vi "Read XML_Parse BC Acyclic Frames.vi"(8 "error in (no error)":errorcluster, 10 "channel in":T1, 11 ".NET Refnum in":refnum<k24>) -> (0 "error out":errorcluster, 2 "channel out":T1, 3 ".NET Refnum out":refnum<k24>)   [LabVIEW 2017, in "Ballard 1553 System Explorer.lvlib"]
uses:
  Ballard 1553 System Explorer.lvlib
  Ballard_Channel.ctl
  Ballard_BC.ctl
  Ballard_message.ctl
  Ballard_messageType.ctl
  Ballard_CWD1.ctl
  Ballard_CWD2.ctl
  Ballard_minorFrame.ctl
  Ballard_majorFrame.ctl
  Ballard_acyclicFrame.ctl
  Ballard_RT.ctl
  Ballard_RT subAddress.ctl
  Ballard_RT direction.ctl
  Ballard_RT rtMode.ctl
  Ballard_RT modeCode.ctl
  D:/Ballard-1553-Custom-Device Inline Async/Source/System Explorer/SubVIs/Parse XML Ballard/Ballard_BTI_XML_Deserializer.dll
  Ballard_BTI_XML_Deserializer.dll
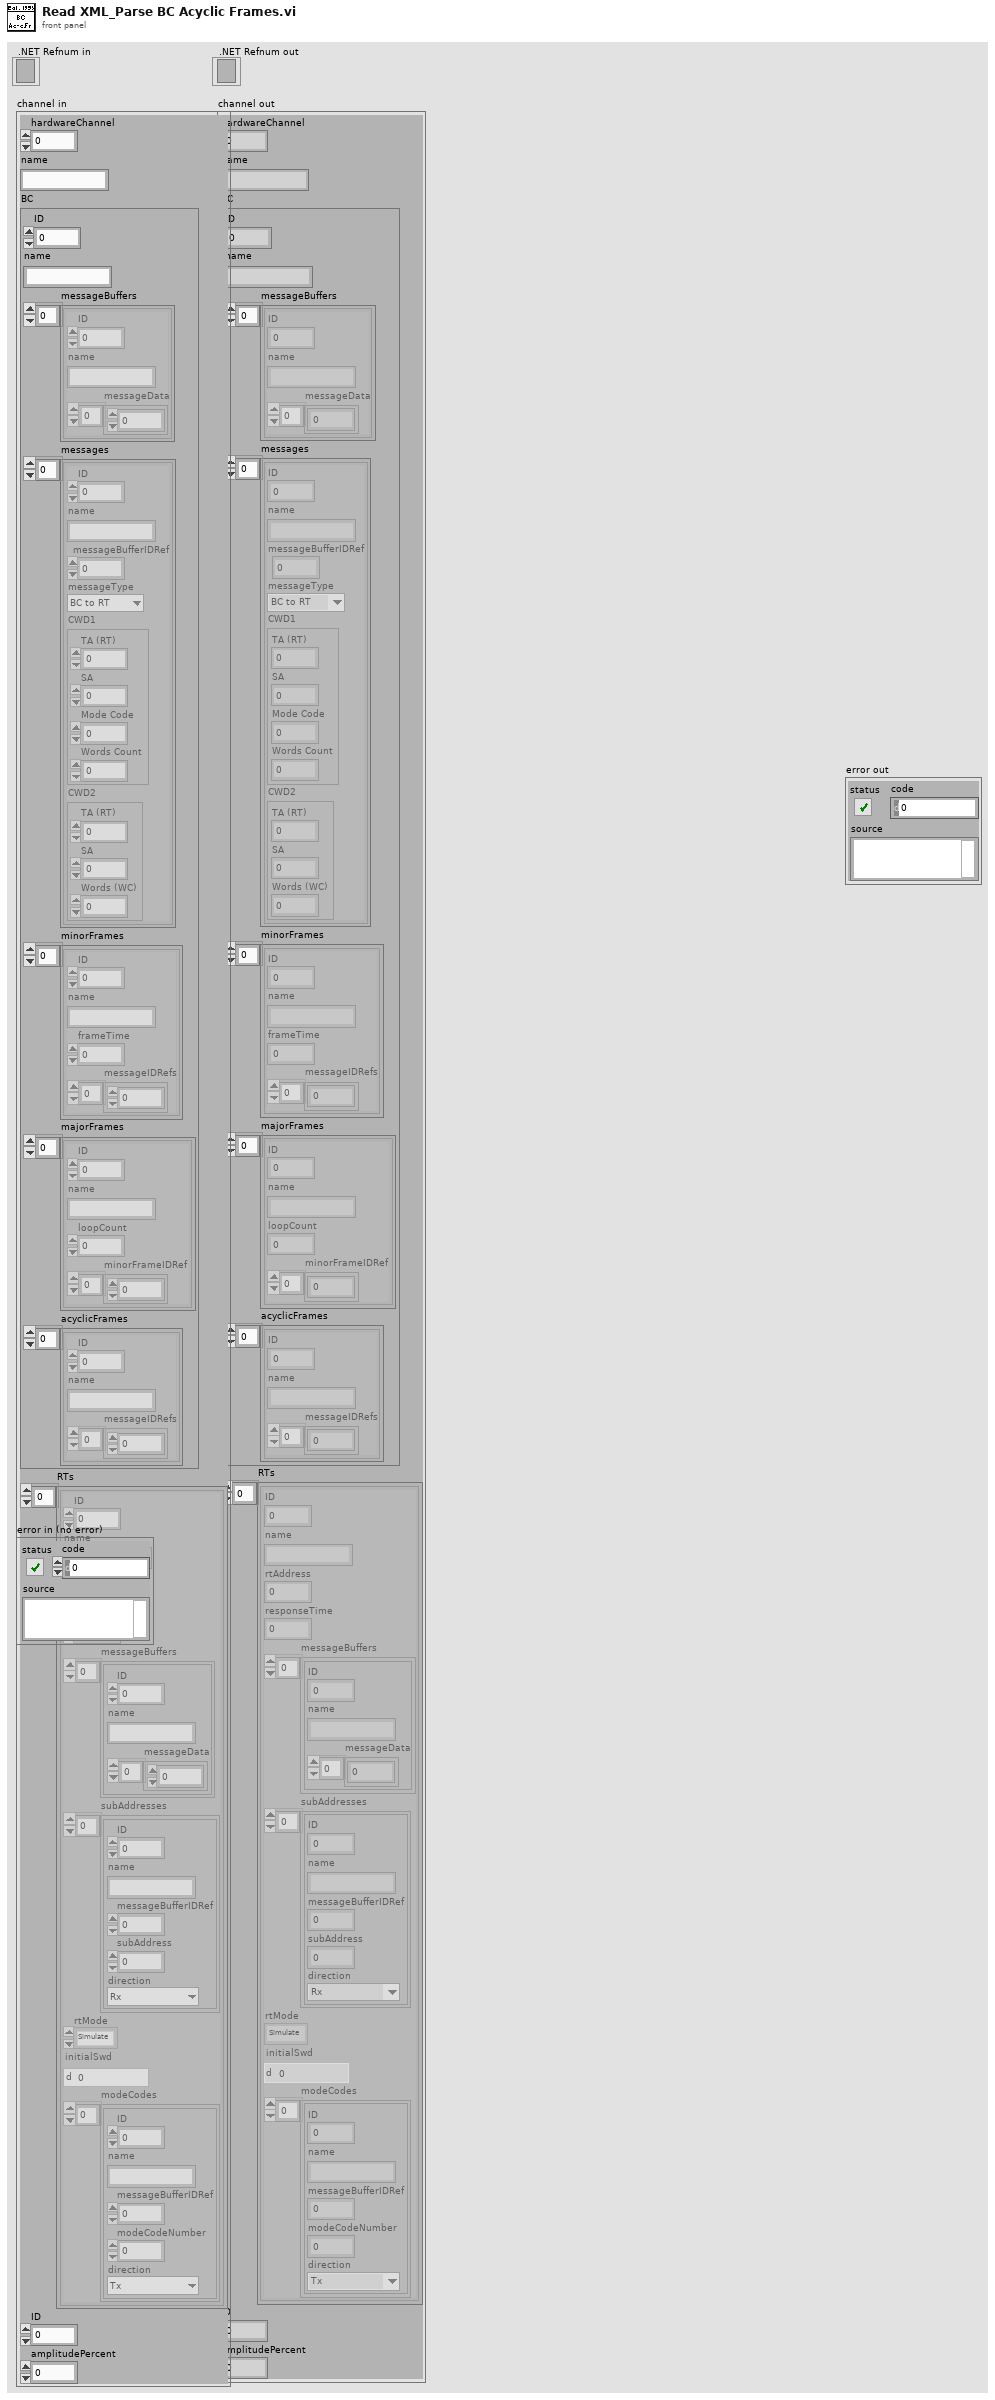
[diagram p1: front panel]
types:
  T1 = typedef "Ballard 1553 System Explorer.lvlib/Ballard_Channel.ctl" = cluster{"hardwareChannel":i32, "name":string, "BC":T2, "RTs":T10[], "ID":i32, "amplitudePercent":dbl}
  T2 = typedef "Ballard 1553 System Explorer.lvlib/Ballard_BC.ctl" = cluster{"ID":i32, "name":string, "messageBuffers":cluster{"ID":i32, "name":string, "messageData":u16[]}[], "messages":T3[], "minorFrames":T7[], "majorFrames":T8[], "acyclicFrames":T9[]}
  T3 = typedef "Ballard 1553 System Explorer.lvlib/Ballard_message.ctl" = cluster{"ID":i32, "name":string, "messageBufferIDRef":i32, "messageType":T4, "CWD1":T5, "CWD2":T6}
  T4 = typedef "Ballard 1553 System Explorer.lvlib/Ballard_messageType.ctl" = enum16{"BC to RT", "RT to BC", "RT to RT", "MC (Rx)", "MC (Tx)"}
  T5 = typedef "Ballard 1553 System Explorer.lvlib/Ballard_CWD1.ctl" = cluster{"TA (RT)":i8, "SA":i8, "Mode Code":i8, "Words Count":i8}
  T6 = typedef "Ballard 1553 System Explorer.lvlib/Ballard_CWD2.ctl" = cluster{"TA (RT)":i8, "SA":i8, "Words (WC)":i8}
  T7 = typedef "Ballard 1553 System Explorer.lvlib/Ballard_minorFrame.ctl" = cluster{"ID":i32, "name":string, "frameTime":i32, "messageIDRefs":i32[]}
  T8 = typedef "Ballard 1553 System Explorer.lvlib/Ballard_majorFrame.ctl" = cluster{"ID":i32, "name":string, "loopCount":i32, "minorFrameIDRef":i32[]}
  T9 = typedef "Ballard 1553 System Explorer.lvlib/Ballard_acyclicFrame.ctl" = cluster{"ID":i32, "name":string, "messageIDRefs":i32[]}
  T10 = typedef "Ballard 1553 System Explorer.lvlib/Ballard_RT.ctl" = cluster{"ID":i32, "name":string, "rtAddress":i8, "responseTime":i32, "messageBuffers":cluster{"ID":i32, "name":string, "messageData":u16[]}[], "subAddresses":T11[], "rtMode":T13, "initialSwd":u16, "modeCodes":T14[]}
  T11 = typedef "Ballard 1553 System Explorer.lvlib/Ballard_RT subAddress.ctl" = cluster{"ID":i32, "name":string, "messageBufferIDRef":i32, "subAddress":i8, "direction":T12}
  T12 = typedef "Ballard 1553 System Explorer.lvlib/Ballard_RT direction.ctl" = enum16{"Tx", "Rx"}
  T13 = typedef "Ballard 1553 System Explorer.lvlib/Ballard_RT rtMode.ctl" = enum16{"Simulate", "Monitor", "Disable"}
  T14 = typedef "Ballard 1553 System Explorer.lvlib/Ballard_RT modeCode.ctl" = cluster{"ID":i32, "name":string, "messageBufferIDRef":i32, "modeCodeNumber":i8, "direction":T12}
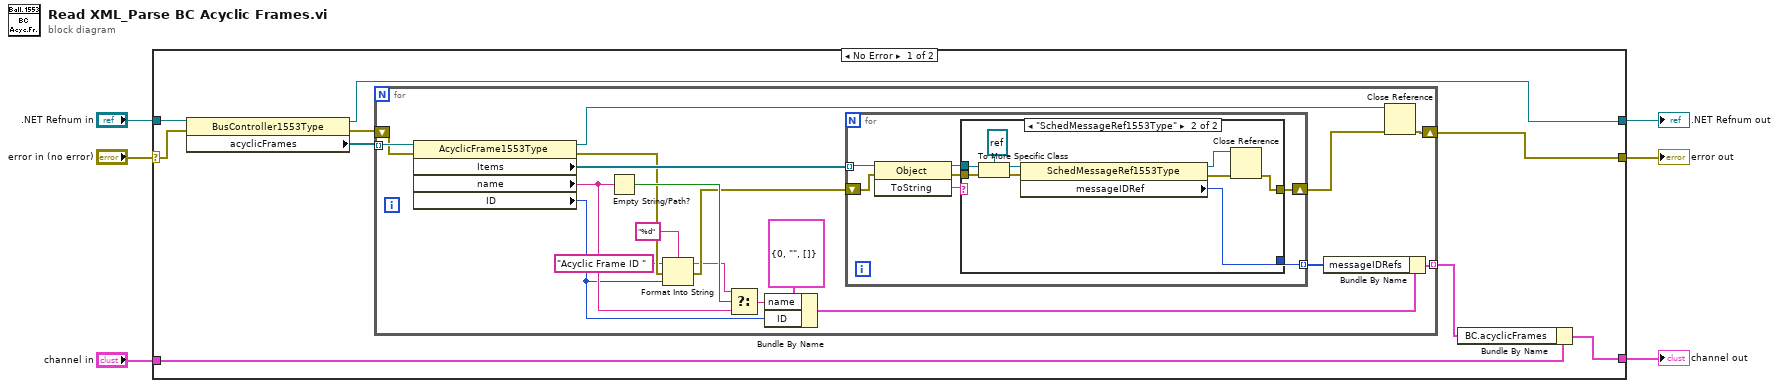
[diagram p0: block diagram]
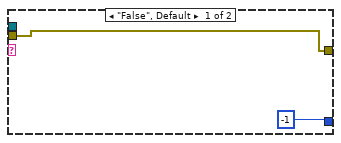
[diagram p2: hidden frame]
diagram:
  n1 = case shown="No Error" "error in (no error)" {
    selector: "error in (no error)" -> [w7 w54]
    tunnel: [w14 w53] -> w6
    tunnel: "channel in" -> [w12 w53]
    tunnel: [w10 w55] -> w4
    tunnel: ".NET Refnum in" -> [w9 w55]
    tunnel: [w8 w54] -> w2
    frame No Error {
      n2 = property class="BusController1553Type"(reference=w9, error in=w7) -> (reference out=w10:refnum<k24>, error out=w15:errorcluster, "acyclicFrames"=w11:refnum<k24>[])
      n3 = for {
        tunnel: w11 -> [w34] mode=indexing
        shift-right: [w31] -> w8
        shift-left: w15 -> [w33]
        tunnel: [w27] -> w13 mode=indexing
        n4 = property class="AcyclicFrame1553Type"(reference=w34, error in=w33) -> (reference out=w32:refnum<k24>, error out=w21:errorcluster, "Items"=w26:refnum<k24>[], "name"=w23:string, "ID"=w19:i32)
        n5 = Empty String/Path?(string/path=w23) -> (empty?=w24:bool)
        n6 = Format Into String(format string="%d", initial string="Acyclic Frame ID ", error in=w21, w19) -> (resulting string=w17:string, error out=w20:errorcluster)
        n7 = Select(t=w17, s=w24, f=w23) -> (s? t:f=w22:string)
        n8 = Bundle By Name(cluster=T9 {"ID"=0, "name"="", "messageIDRefs"=[]} ("acyclicFrame"), "name"=w22, "ID"=w19) -> (w28:T9)
        n9 = for {
          shift-right: [w41] -> w30
          shift-left: w20 -> [w38]
          tunnel: [w40] -> w25 mode=indexing
          tunnel: w26 -> [w39] mode=indexing
          n10 = invoke class="Object" method="ToString"(reference=w39, error in=w38) -> (reference out=w35:refnum<k24>, error out=w36:errorcluster, "ToString"=w37:string)  [unwired: 1 in]
          n11 = case shown="\"SchedMessageRef1553Type\"" w37 {
            tunnel: [w43 w50] -> w41
            tunnel: [-1 ("minorFrameIDRef") w49] -> w40
            tunnel: w36 -> [w43 w45]
            tunnel: w35 -> [_ w48]
            frame "False", Default {
            }
            frame "SchedMessageRef1553Type" {
              n12 = To More Specific Class(target class=refnum<k24> refnum, reference=w48, error in=w45) -> (specific class reference=w47:refnum<k24>, error out=w44:errorcluster)
              n13 = property class="SchedMessageRef1553Type"(reference=w47, error in=w44) -> (reference out=w51:refnum<k24>, error out=w52:errorcluster, "messageIDRef"=w49:i32)
              n14 = Close Reference(reference=w51, error in (no error)=w52) -> (error out=w50:errorcluster)
            }
          }
        }
        n15 = Bundle By Name(cluster=w28, "messageIDRefs"=w25) -> (w27:T9)
        n16 = Close Reference(reference=w32, error in (no error)=w30) -> (error out=w31:errorcluster)
      }
      n17 = Bundle By Name(cluster=w12, "BC.acyclicFrames"=w13) -> (w14:T1)
    }
    frame Error {
    }
  }
  "channel out" <- w6
  ".NET Refnum out" <- w4
  "error out" <- w2
